vi "Box Colour Detection Sequence.vi"() -> (0 "error out":errorcluster, 3 "Colour scan time out?":bool)   [LabVIEW 2018]
uses:
  Modified webcam FGV/Webcam AE.ctl
  <vilib>/userdefined/High Color/IMAQdx.ctl
  Elasped Timer/Elapsed timer control.ctl
panel:
  out "Colour output boolean cluster":T1
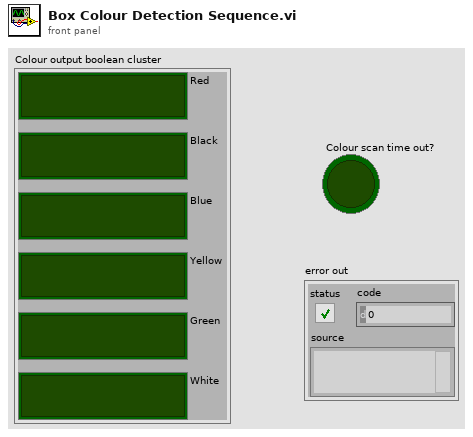
[diagram p1: front panel]
types:
  T1 = cluster{"Red":bool, "Black":bool, "Blue":bool, "Yellow":bool, "Green":bool, "White":bool}
  T2 = typedef "Webcam AE.ctl" = enum16{"Initialize Camera", "Open Camera", "Continuous Acquisition", "Close Camera", "Retrieve Image", "Dispose Camera Image Buffer"}
  T3 = typedef "IMAQdx.ctl" = refnum<k21>
  T4 = typedef "Elapsed timer control.ctl" = enum16{"Start", "Pause", "Initialize"}
  T5 = typedef "IMAQ Image.ctl" = refnum<image>
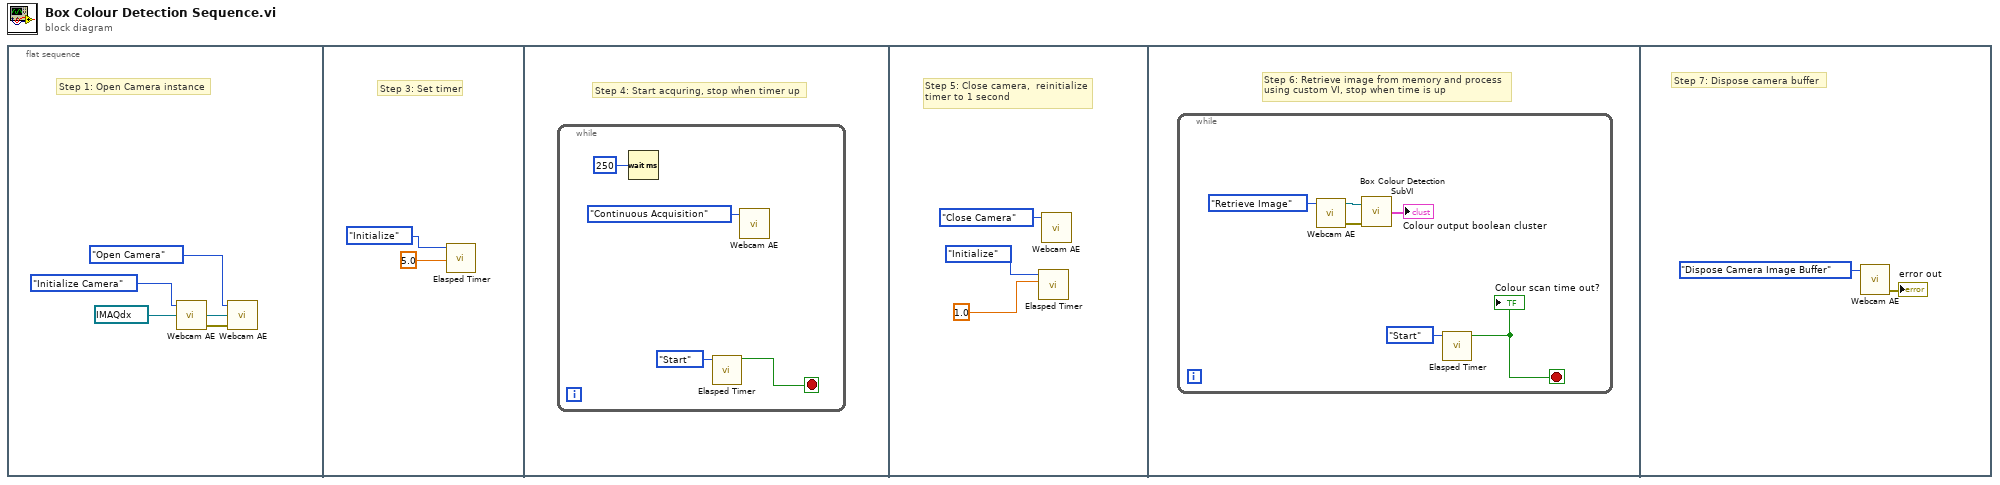
[diagram p0: block diagram]
diagram:
  n1 = flat-sequence {
    frame #0 {
      # "Step 1: Open Camera instance"
      n2 = call "Webcam AE.vi"("Session In"=T3 "cam1", "Camera states"=Webcam_AE."Initialize Camera") -> ("error out"=w4:errorcluster, "Session Out"=w5:T3)  [unwired: 1 in, 1 out]
      n3 = call "Webcam AE.vi"("error in (no error)"=w4, "Session In"=w5, "Camera states"=Webcam_AE."Open Camera") -> ()  [unwired: 3 out]
    }
    frame #1 {
      # "Step 3: Set timer"
      n4 = call "Elasped Timer.vi"("Time Setting"=5.0, "Action"=Elapsed_timer_control."Initialize") -> ()  [unwired: 6 in, 4 out]
    }
    frame #2 {
      # "Step 4: Start acquring, stop when timer up"
      n5 = while {
        stop <- w8 stop-if-true
        n6 = Wait (ms)(milliseconds to wait=u32 250 ("millisecond timer value")) -> ()  [unwired: 1 out]
        n7 = call "Elasped Timer.vi"("Action"=Elapsed_timer_control."Start") -> ("Time Out?!"=w8:bool)  [unwired: 7 in, 3 out]
        n8 = call "Webcam AE.vi"("Camera states"=Webcam_AE."Continuous Acquisition") -> ()  [unwired: 2 in, 3 out]
      }
    }
    frame #3 {
      # "Step 5: Close camera,  reinitialize \ntimer to 1 second"
      n9 = call "Elasped Timer.vi"("Time Setting"=1.0, "Action"=Elapsed_timer_control."Initialize") -> ()  [unwired: 6 in, 4 out]
      n10 = call "Webcam AE.vi"("Camera states"=Webcam_AE."Close Camera") -> ()  [unwired: 2 in, 3 out]
    }
    frame #4 {
      # "Step 6: Retrieve image from memory and process\nusing custom VI, stop when time is up"
      n11 = while {
        stop <- w15 stop-if-true
        n12 = call "Webcam AE.vi"("Camera states"=Webcam_AE."Retrieve Image") -> ("error out"=w17:errorcluster, "Image Out"=w18:T5)  [unwired: 2 in, 1 out]
        n13 = call "Box Colour Detection SubVI.vi"("Image In"=w18, "Error In"=w17) -> ("Colour output boolean cluster"=→"Colour output boolean cluster":T1)  [unwired: 2 out]
        n14 = call "Elasped Timer.vi"("Action"=Elapsed_timer_control."Start") -> ("Time Out?!"=w15:bool)  [unwired: 7 in, 3 out]
        "Colour scan time out?" <- w15
      }
    }
    frame #5 {
      # "Step 7: Dispose camera buffer"
      n15 = call "Webcam AE.vi"("Camera states"=Webcam_AE."Dispose Camera Image Buffer") -> ("error out"=→"error out":errorcluster)  [unwired: 2 in, 2 out]
    }
  }
